vi "getCE_ExpPath.vi"   [LabVIEW 2019]
uses:
  <userlib>/LevyLab/Transport/Control Experiment/Control Experiment.lvclass
  <vilib>/Wiresmith Technology/G CLI/CLI Class/CLI.lvclass
panel:
  # "[FLEX <-> getExpPath] \nThis VI calls VNA.vi upon a terminal command\ncommand: g-cli --lv-ver 2019 <path of the vi>"
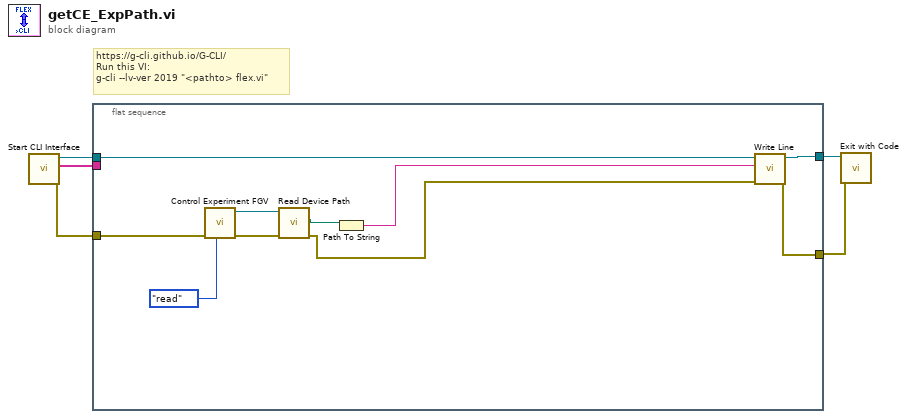
[diagram p0: block diagram]
diagram:
  # "https://g-cli.github.io/G-CLI/\nRun this VI:\ng-cli --lv-ver 2019 \"<pathto> flex.vi\""
  n1 = call <vilib>:"Start CLI Interface.vi"() -> ("error out"=w5:errorcluster, "Custom Parameters"=w1:string[], "CLI out"=w4:refnum<class "CLI.lvclass">)  [unwired: 8 in, 1 out]
  n2 = flat-sequence {
    tunnel: w5 -> [w10]
    tunnel: w4 -> [w15]
    tunnel: [w14] -> w3
    tunnel: [w13] -> w2
    tunnel: w1 -> [_]
    frame #0 {
      n3 = call <userlib>:"Control Experiment FGV.vi"("Function"=enum16{"read", "write"}."read", "error in (no error)"=w10) -> ("error out"=w7:errorcluster, "Control Experiment.lvclass out"=w9:refnum<class "Control Experiment.lvclass">)  [unwired: 8 in]
      n4 = call <userlib>:"Read Device Path.vi"("error in (no error)"=w7, "Control Experiment in"=w9) -> ("error out"=w6:errorcluster, "Device Path"=w8:path)  [unwired: 7 in, 1 out]
      n5 = Path To String(path=w8) -> (string=w12:string)
      n6 = call <vilib>:"Write Line.vi"("error in (no error)"=w6, "Text to Write"=w12, "CLI in"=w15) -> ("error out"=w13:errorcluster, "CLI out"=w14:refnum<class "CLI.lvclass">)  [unwired: 7 in]
    }
  }
  n7 = call <vilib>:"Exit with Code.vi"("error in (no error)"=w2, "CLI in"=w3) -> ()  [unwired: 9 in, 1 out]
